vi "UDP Communication.vi"(8 "error out":errorcluster) -> ()   [LabVIEW 2013]
uses:
  UDP Dashboard Packet.ctl
  Autonomous Setpoints.ctl
  Auto Shift Settings.ctl
  Shoot Profile.ctl
  Halo Drive.ctl
  Auto Speed Constants.ctl
  Autonomous Center Line Setpoints.ctl
  Robot Global Data.vi
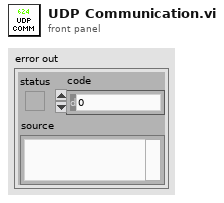
[diagram p1: front panel]
types:
  T1 = typedef "UDP Dashboard Packet.ctl" = cluster{"Feed Angle":dbl, "Neutral Angle":dbl, "Autonomous Setpoints":T2, "Auto Shift":T3, "Elevator Angle Offset":dbl, "Potentiometer Angle":cluster{"Pot M":dbl, "Pot B":dbl}, "Shoot Setpoints":cluster{"Vision":T4, "Back Corner":T4, "Front":T4, "Front Corner":T4, "Half Court":T4, "Full Court":T4, "Pyramid":T4}, "Halo Drive":T5, "Auto Speed Constants":T6, "Shooting Delays":cluster{"Unjam On":dbl, "Unjam Off":dbl, "Flipper On":dbl, "Flipper Off":dbl, "Hopper Up":dbl}, "Left Roller Pwr":dbl, "Right Roller Pwr":dbl, "Elevator PID Gains":cluster{"proportional gain (Kc)":dbl, "integral time (Ti, min)":dbl, "derivative time (Td, min)":dbl}, "Elevator PID Output Range":cluster{"output high":dbl, "output low":dbl}, "Elevator Angle Tolerance":dbl, "Toggle Ears Delay":dbl, "Toggle Ears Distance":dbl, "Unjam Servo Angle":dbl, "Auton Steer PID gains":cluster{"proportional gain (Kc)":dbl, "integral time (Ti, min)":dbl, "derivative time (Td, min)":dbl}, "Auton Steer output range":cluster{"output high":dbl, "output low":dbl}, "Auto Reverse Speed":dbl, "Auto Stop Throttle":dbl, "Auto Stop Duration":dbl, "Spin output range":cluster{"output high":dbl, "output low":dbl}, "Spin PID gains":cluster{"proportional gain (Kc)":dbl, "integral time (Ti, min)":dbl, "derivative time (Td, min)":dbl}, "Auto-Center Line":T7, "Auton Distance PID gains Low Gear":cluster{"proportional gain (Kc)":dbl, "integral time (Ti, min)":dbl, "derivative time (Td, min)":dbl}, "Auton Distance output range":cluster{"output high":dbl, "output low":dbl}, "Auton Distance Threshold":dbl, "Auton Velocity Cutoff":dbl, "Auton Distance output range Center Line":cluster{"output high":dbl, "output low":dbl}, "Auton Distance PID gains High Gear":cluster{"proportional gain (Kc)":dbl, "integral time (Ti, min)":dbl, "derivative time (Td, min)":dbl}}
  T2 = typedef "Autonomous Setpoints.ctl" = cluster{"Shoot Angle 1":dbl, "Initial Delay":dbl, "Disc Count 1":dbl, "Shoot Time 1":dbl, "Distance 1":dbl, "Two Disc Distance 1":dbl, "Distance 2":dbl, "Two Disc Distance 2":dbl, "Distance 3":dbl, "Two Disc Distance 3":dbl, "Shoot Angle 3":dbl, "Disc Count 3":dbl, "Shoot Time 3":dbl, "Distance 4":dbl, "Two Disc Distance 4":dbl, "Low Gear":bool, "Shoot 1 Post Delay":dbl}
  T3 = typedef "Auto Shift Settings.ctl" = cluster{"Enabled":bool, "Upshift Speed":dbl, "Downshift Speed":dbl, "Upshift Throttle":dbl, "Turn Power Diff":dbl, "Motor Limit":dbl, "Encoder Limit":dbl}
  T4 = typedef "Shoot Profile.ctl" = cluster{"Pre RPM":dbl, "Main RPM":dbl, "Angle":dbl}
  T5 = typedef "Halo Drive.ctl" = cluster{"Gains":cluster{"Quickturn_Sens_Low":dbl, "Quickturn_Sens_High":dbl, "Speedturn_Sens_Low":dbl, "Speedturn_Sens_High":dbl}, "QuickTurn Const":dbl, "Loading Throttle Limit":dbl}
  T6 = typedef "Auto Speed Constants.ctl" = cluster{"Slowing Distance":dbl, "High Speed":dbl, "Rampup Time":dbl, "Low Speed":dbl, "High Speed (Reverse)":dbl}
  T7 = typedef "Autonomous Center Line Setpoints.ctl" = cluster{"Arc Turn x-axis":dbl, "Arc Turn y-axis":dbl, "Arc Turn Distance":dbl, "Distance 1":dbl, "Two Disc Distance 1":dbl, "Distance 2":dbl, "Two Disc Distance 2":dbl, "Spin Angle":dbl, "Spin Angle tolerance":dbl, "Spin y-axis":dbl, "Spin Distance":dbl, "Center Line Enabled":bool, "Distance 3":dbl, "Two Disc Distance 3":dbl, "Spin Angle 2":dbl, "Spin Angle tolerance 2":dbl, "Spin y-axis 2":dbl, "Spin Distance 2":dbl, "Shoot Angle 1":dbl, "Disc Count 1":dbl, "Shoot Time 1":dbl, "Shoot Angle 3":dbl, "Disc Count 3":dbl, "Shoot Time 3":dbl, "Low Gear":bool}
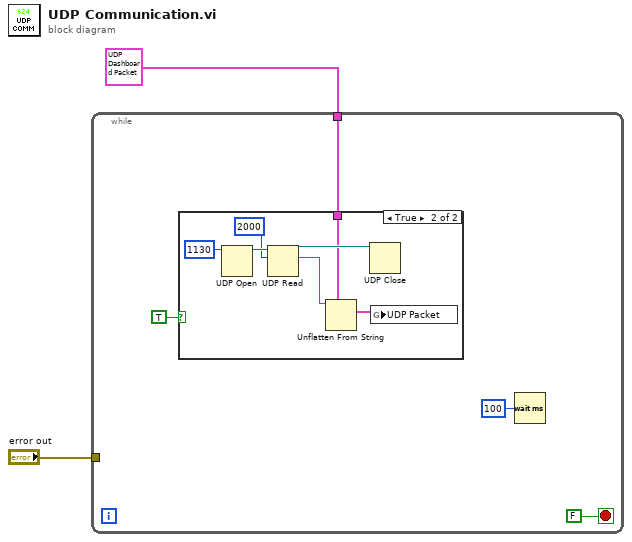
[diagram p0: block diagram]
diagram:
  n1 = while {
    tunnel: T1 {"Feed Angle"=3500.0, "Neutral Angle"=4000.0, "Autonomous Setpoints"={"Shoot Angle 1"=3500.0, "Initial Delay"=4000.0, "Disc Count 1"=27.0, "Shoot Time 1"=0.0, "Distance 1"=0.0, "Two Disc Distance 1"=0.0, "Distance 2"=0.0, "Two Disc Distance 2"=0.0, "Distance 3"=0.0, "Two Disc Distance 3"=0.0, "Shoot Angle 3"=0.0, "Disc Count 3"=0.0, "Shoot Time 3"=0.0, "Distance 4"=0.0, "Two Disc Distance 4"=0.0, "Low Gear"=FALSE, "Shoot 1 Post Delay"=0.0}, "Auto Shift"={"Enabled"=FALSE, "Upshift Speed"=4000.0, "Downshift Speed"=27.0, "Upshift Throttle"=0.0, "Turn Power Diff"=0.0, "Motor Limit"=0.0, "Encoder Limit"=0.0}, "Elevator Angle Offset"=0.0, "Potentiometer Angle"={"Pot M"=0.0, "Pot B"=0.0}, "Shoot Setpoints"={"Vision"={"Pre RPM"=0.0, "Main RPM"=0.0, "Angle"=0.0}, "Back Corner"={"Pre RPM"=0.0, "Main RPM"=0.0, "Angle"=0.0}, "Front"={"Pre RPM"=0.0, "Main RPM"=0.0, "Angle"=0.0}, "Front Corner"={"Pre RPM"=0.0, "Main RPM"=0.0, "Angle"=0.0}, "Half Court"={"Pre RPM"=0.0, "Main RPM"=0.0, "Angle"=0.0}, "Full Court"={"Pre RPM"=0.0, "Main RPM"=0.0, "Angle"=0.0}, "Pyramid"={"Pre RPM"=0.0, "Main RPM"=0.0, "Angle"=0.0}}, "Halo Drive"={"Gains"={"Quickturn_Sens_Low"=0.0, "Quickturn_Sens_High"=0.0, "Speedturn_Sens_Low"=0.0, "Speedturn_Sens_High"=0.0}, "QuickTurn Const"=0.0, "Loading Throttle Limit"=0.0}, "Auto Speed Constants"={"Slowing Distance"=0.0, "High Speed"=0.0, "Rampup Time"=0.0, "Low Speed"=0.0, "High Speed (Reverse)"=0.0}, "Shooting Delays"={"Unjam On"=0.0, "Unjam Off"=0.0, "Flipper On"=0.0, "Flipper Off"=0.0, "Hopper Up"=0.0}, "Left Roller Pwr"=0.0, "Right Roller Pwr"=0.0, "Elevator PID Gains"={"proportional gain (Kc)"=0.0, "integral time (Ti, min)"=0.0, "derivative time (Td, min)"=0.0}, "Elevator PID Output Range"={"output high"=0.0, "output low"=0.0}, "Elevator Angle Tolerance"=0.0, "Toggle Ears Delay"=0.0, "Toggle Ears Distance"=0.0, "Unjam Servo Angle"=0.0, "Auton Steer PID gains"={"proportional gain (Kc)"=0.0, "integral time (Ti, min)"=0.0, "derivative time (Td, min)"=0.0}, "Auton Steer output range"={"output high"=0.0, "output low"=0.0}, "Auto Reverse Speed"=0.0, "Auto Stop Throttle"=0.0, "Auto Stop Duration"=0.0, "Spin output range"={"output high"=0.0, "output low"=0.0}, "Spin PID gains"={"proportional gain (Kc)"=0.0, "integral time (Ti, min)"=0.0, "derivative time (Td, min)"=0.0}, "Auto-Center Line"={"Arc Turn x-axis"=0.0, "Arc Turn y-axis"=0.0, "Arc Turn Distance"=0.0, "Distance 1"=0.0, "Two Disc Distance 1"=0.0, "Distance 2"=0.0, "Two Disc Distance 2"=0.0, "Spin Angle"=0.0, "Spin Angle tolerance"=0.0, "Spin y-axis"=0.0, "Spin Distance"=0.0, "Center Line Enabled"=FALSE, "Distance 3"=0.0, "Two Disc Distance 3"=0.0, "Spin Angle 2"=0.0, "Spin Angle tolerance 2"=0.0, "Spin y-axis 2"=0.0, "Spin Distance 2"=0.0, "Shoot Angle 1"=0.0, "Disc Count 1"=0.0, "Shoot Time 1"=0.0, "Shoot Angle 3"=0.0, "Disc Count 3"=0.0, "Shoot Time 3"=0.0, "Low Gear"=FALSE}, "Auton Distance PID gains Low Gear"={"proportional gain (Kc)"=0.0, "integral time (Ti, min)"=0.0, "derivative time (Td, min)"=0.0}, "Auton Distance output range"={"output high"=0.0, "output low"=0.0}, "Auton Distance Threshold"=0.0, "Auton Velocity Cutoff"=0.0, "Auton Distance output range Center Line"={"output high"=0.0, "output low"=0.0}, "Auton Distance PID gains High Gear"={"proportional gain (Kc)"=0.0, "integral time (Ti, min)"=0.0, "derivative time (Td, min)"=0.0}} ("UDP Packet") -> [w6]
    tunnel: "error out" -> [_]
    stop <- FALSE stop-if-true
    n2 = case shown="True" TRUE {
      tunnel: w6 -> [_ w10]
      frame False {
      }
      frame True {
        n3 = UDP Open(11:u16 1130 ("port")) -> (port=w13:refnum<k16>)  [unwired: 4 in, 2 out]
        n4 = UDP Read(connection ID=w13, max size (548)=2000) -> (data out=w11:string, 3:w12:refnum<k16>)  [unwired: 2 in, 3 out]
        n5 = Unflatten From String(type=w10, binary string=w11) -> (value=w8:T1)  [unwired: 3 in, 2 out]
        n6 = UDP Close(connection ID=w12) -> ()  [unwired: 1 in, 2 out]
        n7 = global write "Robot Global Data.vi" "UDP Packet"(w8) -> ()
      }
    }
    n8 = Wait (ms)(milliseconds to wait=u32 100) -> ()  [unwired: 1 out]
  }
